vi "MotorRotate.vi"(2 "角度":dbl, 3 "axis":i32) -> (1 "返回":i32)   [LabVIEW 2018]
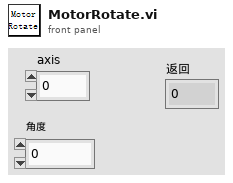
[diagram p1: front panel]
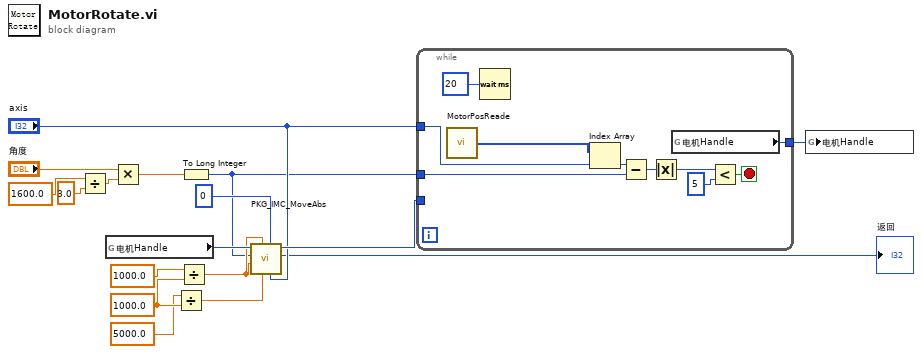
[diagram p0: block diagram]
diagram:
  w9 = 1000.0 ("y")
  n1 = Divide(x=1600.0, y=3.0) -> (x/y=w13:dbl)
  n2 = global read "参数.vi" "电机Handle"() -> (w11:u32)
  n3 = Multiply(x="角度", y=w13) -> (x*y=w12:dbl)
  n4 = Divide(x=5000.0, y=w9) -> (x/y=w7:dbl)
  n5 = Divide(x=1000.0, y=w9) -> (x/y=w6:dbl)
  n6 = To Long Integer(number=w12) -> (32bit integer=w3:i32)
  n7 = call "PKG_IMC_MoveAbs.vi"("axis"="axis", "wait"=0, "tgvel"=w7, "endvel"=w6, "startvel"=w6, "pos"=w3, "handle"=w11) -> ("function return"=→"返回":i32, "handle out"=w5:u32)  [unwired: 3 in]
  n8 = while {
    tunnel: w5 -> [_]
    tunnel: "axis" -> [w25]
    tunnel: w3 -> [w23]
    tunnel: [w18] -> w2
    stop <- w19 stop-if-true
    n9 = call "MotorPosReade.vi"() -> ("坐标输出"=w26:i32[])  [unwired: 1 in]
    n10 = Wait (ms)(milliseconds to wait=u32 20 ("等待时间（毫秒）")) -> ()  [unwired: 1 out]
    n11 = Index Array(array=w26, index=w25) -> (element=w24:i32)
    n12 = Subtract(x=w24, y=w23) -> (x-y=w22:i32)
    n13 = Absolute Value(x=w22) -> (abs(x)=w21:i32)
    n14 = global read "参数.vi" "电机Handle"() -> (w18:u32)
    n15 = Less?(x=w21, y=5) -> (x < y?=w19:bool)
  }
  n16 = global write "参数.vi" "电机Handle"(w2) -> ()
